vi "date acq.vi"() -> ()   [LabVIEW 2013]
panel:
  out "substring before match":string
  in  "date format (0)":enum16{"short", "long", "abbreviated"}(ring)
  out "time string":string
  out "date string":string
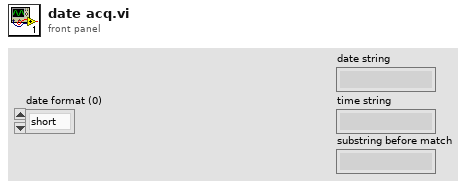
[diagram p1: front panel]
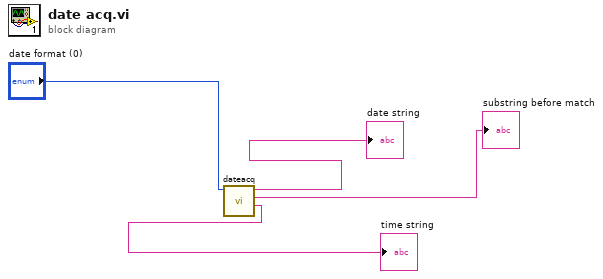
[diagram p0: block diagram]
diagram:
  n1 = call "dateacq.vi"("date format (0)"="date format (0)") -> ("time string"=→"time string":string, "substring before match"=→"substring before match":string, "date string"=→"date string":string)  [unwired: 8 in]
